vi "Cannon Global Data.vi"() -> ()   [LabVIEW 2012]
panel:
  in  "Stop Comprerssor?":bool
  in  "Cannon Information":T1
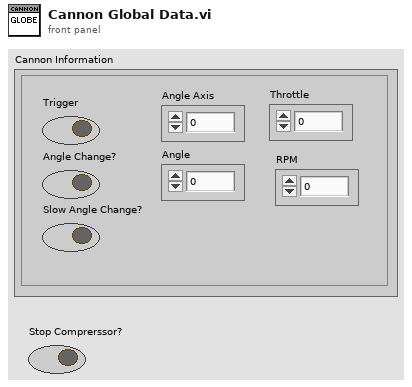
[diagram p1: front panel]
types:
  T1 = cluster{"RPM":dbl, "Trigger":bool, "Angle Axis":dbl, "Angle":dbl, "Throttle":dbl, "Slow Angle Change?":bool, "Angle Change?":bool}
diagram:
